vi "Initialise State.vi"(8 "error in (no error)":errorcluster, 11 "OnChange_Boolean in":refnum<class "OnChangeNotifier_U64.lvclass">) -> (0 "error out":errorcluster, 3 "OnChange_Boolean out":refnum<class "OnChangeNotifier_U64.lvclass">)   [LabVIEW 2021, in "OnChangeNotifier_U64.lvclass"]
uses:
  OnChangeNotifier_U64.lvclass
  <vilib>/TSA/Abstract Data Classes/Abs_Types/U32 Integer/Static Read.vi
  <vilib>/TSA/Abstract Data Classes/Abs_Types/U32 Integer/Abs_U32 Integer.lvclass
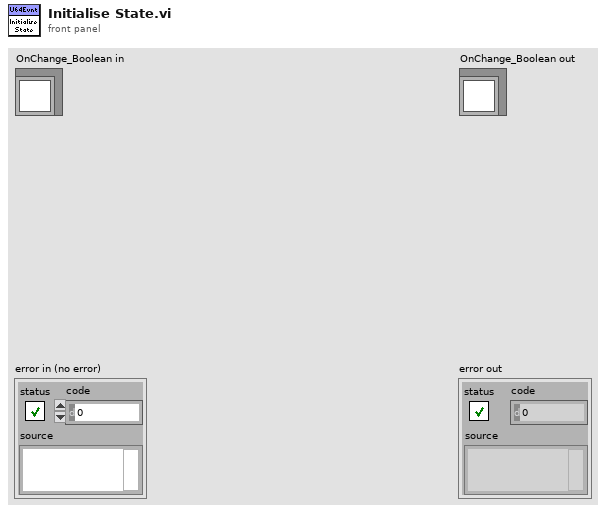
[diagram p1: front panel]
types:
  T1 = typedef "OnChangeNotifier_U64.lvclass/Class Type.ctl" = refnum<class "Abs_U32 Integer.lvclass">
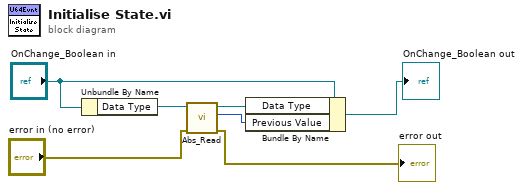
[diagram p0: block diagram]
diagram:
  n1 = Unbundle By Name("OnChange_Boolean in") -> ("Data Type"=w7:T1)
  n2 = call-poly <vilib>:"Abs_Read.vi"("error in (no error)"="error in (no error)", "Abs_U32 Integer in"=w7) -> ("error out"=→"error out":errorcluster, "Value"=w3:u32, "Abs_U32 Integer out"=w5:T1)  [unwired: 7 in]
  n3 = Bundle By Name(cluster="OnChange_Boolean in", "Data Type"=w5, "Previous Value"=w3) -> (→"OnChange_Boolean out":refnum<class "OnChangeNotifier_U64.lvclass">)
